vi "Tag_settings_save.vi"(8 "error in (no error)":errorcluster, 9 "PresetSave":T1 {"Presets"."max" format="%#_3p"; "Presets"."min" format="%#_3p"}, 11 "Gviewer in":refnum<class "Gviewer.lvclass">) -> (0 "error out":errorcluster, 3 "Gviewer out":refnum<class "Gviewer.lvclass">)   [LabVIEW 2020, in "Gviewer.lvclass"]
doc: "Andre Koelewijn, 5 feb 2021\n\nSave presets from one of the Viewports"
uses:
  Gviewer.lvclass
  controls/Typedef_PresetSave.ctl
  controls/EditTagOneTag.ctl
  controls/Typedef-PresetFileFormat.ctl
  Gviewer.lvclass/Gviewer.ctl
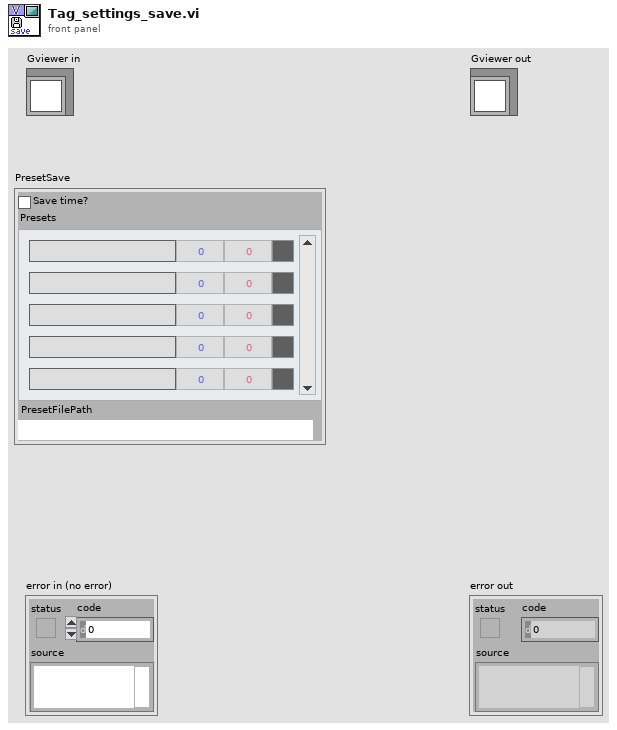
[diagram p1: front panel]
types:
  T1 = typedef "Gviewer.lvclass/Typedef_PresetSave.ctl" = cluster{"Save time?":bool, "Presets":T2[], "PresetFilePath":path}
  T2 = typedef "Gviewer.lvclass/EditTagOneTag.ctl" = cluster{"TAG":string, "min":dbl, "max":dbl, "Color":u32}
  T3 = enum16{"big-endian, network order", "native, host order", "little-endian"}
  T4 = typedef "Gviewer.lvclass/Typedef-PresetFileFormat.ctl" = cluster{"Time-Start":timestamp, "Time-End":timestamp, "Time-File":timestamp, "PresetSave":cluster{"Save time?":bool, "Presets":T2[], "PresetFilePath":path}}
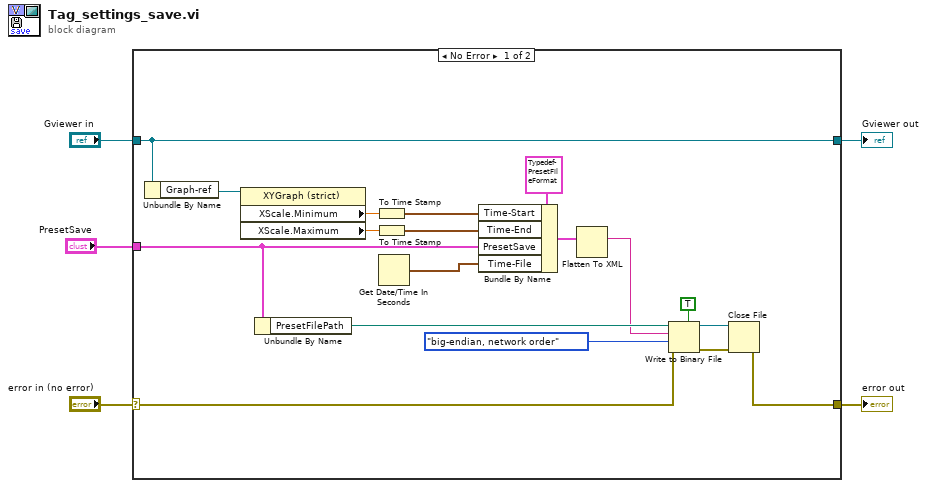
[diagram p0: block diagram]
diagram:
  n1 = case shown="No Error" "error in (no error)" {
    selector: "error in (no error)" -> [w9 w25]
    tunnel: [w6 w25] -> w4
    tunnel: [w23 w24] -> w2
    tunnel: "Gviewer in" -> [w23 w24]
    tunnel: "PresetSave" -> [w14 _]
    frame No Error {
      n2 = Unbundle By Name(w23) -> ("Graph-ref"=w21:refnum<vi>)
      n3 = property class="XYGraph (strict)"(reference=w21) -> ("XScale.Minimum"=w20:dbl, "XScale.Maximum"=w19:dbl)  [unwired: 1 in, 2 out]
      n4 = Unbundle By Name(w14) -> ("PresetFilePath"=w13:path)
      n5 = To Time Stamp(1:w20) -> (0:w18:timestamp)
      n6 = To Time Stamp(1:w19) -> (0:w17:timestamp)
      n7 = Get Date/Time In Seconds() -> (seconds since 1Jan1904=w16:timestamp)
      n8 = Bundle By Name(cluster=T4 {"Time-Start"=timestamp(0 s since 1904-01-01), "Time-End"=timestamp(0 s since 1904-01-01), "Time-File"=timestamp(0 s since 1904-01-01), "PresetSave"={"Save time?"=FALSE, "Presets"=[], "PresetFilePath"=path ""}} ("PresetFileFormat"), "Time-Start"=w18, "Time-End"=w17, "PresetSave"=w14, "Time-File"=w16) -> (w15:T4)
      n9 = Flatten To XML(6:w15) -> (2:w11:string)
      n10 = Write to Binary File(file (use dialog)=w13, data=w11, error in=w9, 5:TRUE ("prepend array or string size? (T)"), 9:T3."big-endian, network order" ("byte order (0:big-endian, network order)")) -> (refnum out=w8:refnum<file>, error out=w7:errorcluster)  [unwired: 1 in, 1 out]
      n11 = Close File(refnum=w8, error in=w7) -> (error out=w6:errorcluster)  [unwired: 1 out]
    }
    frame Error {
    }
  }
  "error out" <- w4
  "Gviewer out" <- w2
